vi "Write Chirp.vi"(8 "error in (no error)":errorcluster, 10 "Chirp":cluster{"f_center":dbl, "bandwidth":dbl}={"f_center"=1350.0, "bandwidth"=150.0}, 11 "PAS in":refnum<class "PAS.lvclass">) -> (0 "error out":errorcluster, 3 "PAS out":refnum<class "PAS.lvclass">)   [LabVIEW 2015, in "PAS.lvclass"]
uses:
  PAS.lvclass
  PAS.lvclass/PAS.ctl
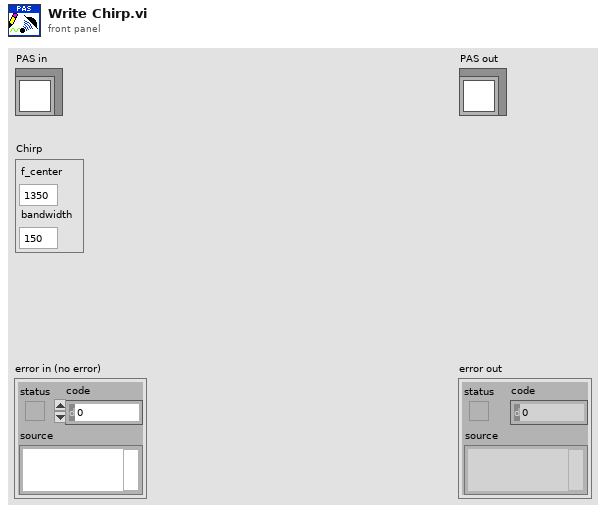
[diagram p1: front panel]
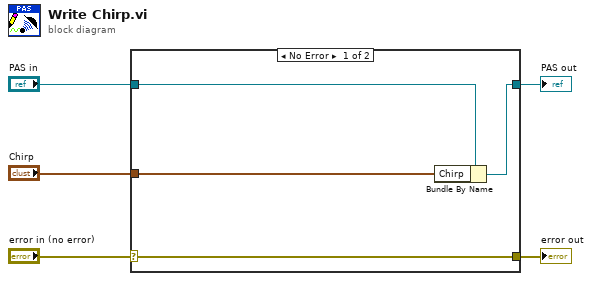
[diagram p0: block diagram]
diagram:
  n1 = case shown="No Error" "error in (no error)" {
    selector: "error in (no error)" -> [w9 w10]
    tunnel: [w9 w10] -> w4
    tunnel: [w7 w11] -> w2
    tunnel: "PAS in" -> [w8 w11]
    tunnel: "Chirp" -> [w6 _]
    frame No Error {
      n2 = Bundle By Name(cluster=w8, "Chirp"=w6) -> (w7:refnum<class "PAS.lvclass">)
    }
    frame Error {
    }
  }
  "error out" <- w4
  "PAS out" <- w2
